vi "ReversedEngineering SortTypeDefsInOrder.vi"(1 "Types":T1(array[cluster])) -> (15 "TypesOut":T1(array[cluster]))   [LabVIEW 2016]
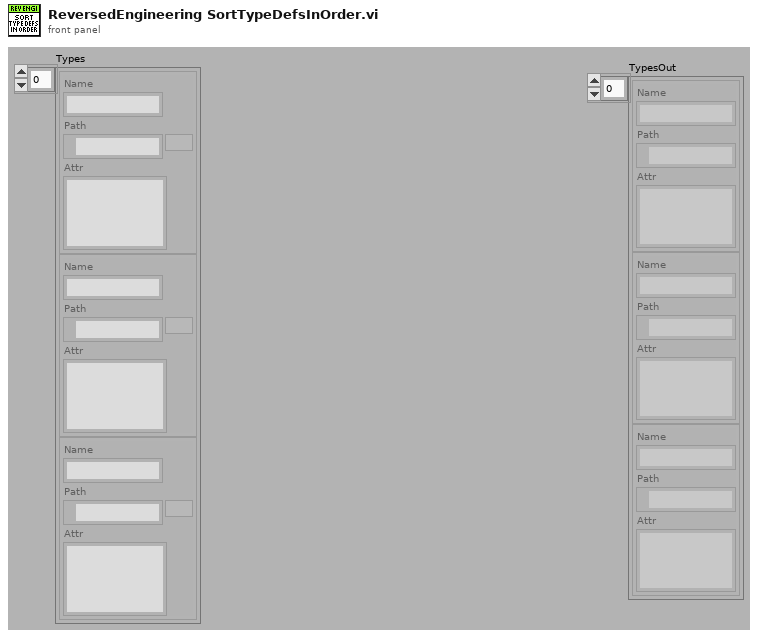
[diagram p1: front panel]
types:
  T1 = cluster{"Name":string, "Path":path, "Attr":string}[]
  T2 = cluster{"Name":string, "Path":path, "Attr":string}
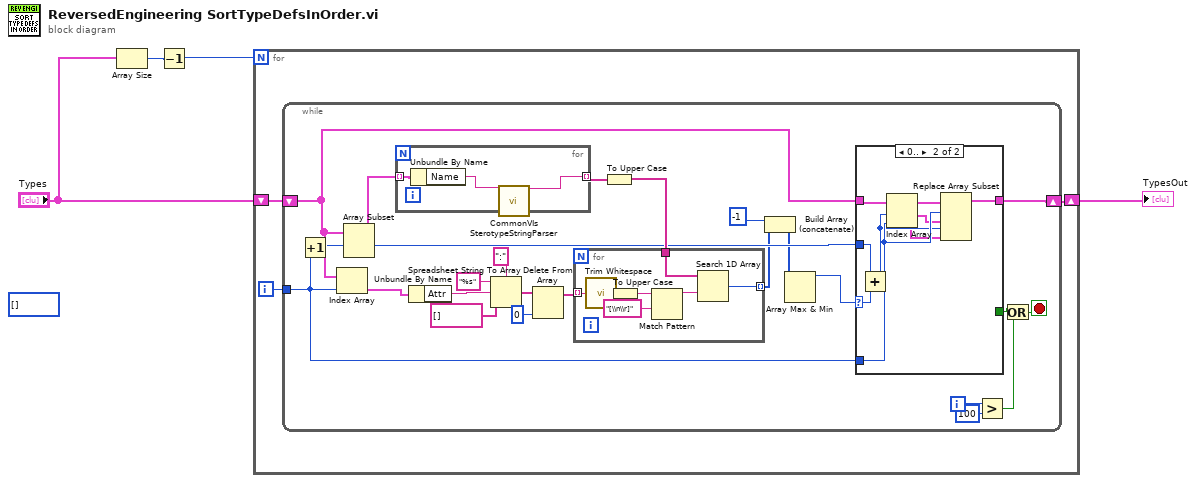
[diagram p0: block diagram]
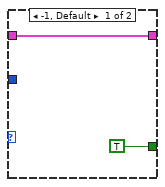
[diagram p2: hidden frame]
diagram:
  (unwired) i32[] []
  n1 = Array Size(array="Types") -> (size(s)=w2:i32)
  n2 = Decrement(x=w2) -> (x-1=w1:i32)
  n3 = for {
    N: w1 -> [_]
    shift-right: [w5] -> w4
    shift-left: "Types" -> [w6]
    i -> [w7]
    n4 = while {
      tunnel: w7 -> [w13]
      shift-right: [w20] -> w5
      shift-left: w6 -> [w19]
      i -> [w17]
      stop <- w15 stop-if-true
      n5 = Increment(x=w13) -> (x+1=w12:i32)
      n6 = Index Array(array=w19, index=w13) -> (element=w21:T2)
      n7 = Array Subset(array=w19, index=w12) -> (w22:T1)  [unwired: 1 in]
      n8 = for {
        tunnel: w22 -> [w44] mode=indexing
        tunnel: [w42] -> w27 mode=indexing
        n9 = Unbundle By Name(w44) -> ("Name"=w43:string)
        n10 = call <resource>:"CommonVIs SterotypeStringParser.vi"("SterotypeStringIn"=w43) -> ("Name"=w42:string)  [unwired: 18 out]
      }
      n11 = Unbundle By Name(w21) -> ("Attr"=w31:string)
      n12 = Spreadsheet String To Array(delimiter (Tab)=":", format string="%s", spreadsheet string=w31, array type (2D Dbl)=string[] []) -> (array=w25:string[])
      n13 = Delete From Array(array=w25, index=0) -> (array with subset deleted=w24:string[])  [unwired: 1 in, 1 out]
      n14 = To Upper Case(1:w27) -> (0:w26:string[])
      n15 = for {
        tunnel: w24 -> [w51] mode=indexing
        tunnel: w26 -> [w47]
        tunnel: [w45] -> w9 mode=indexing
        n16 = call <vilib>:"Trim Whitespace.vi"("string"=w51) -> ("trimmed string"=w46:string)  [unwired: 1 in]
        n17 = To Upper Case(1:w46) -> (0:w50:string)
        n18 = Match Pattern(string=w50, regular expression="[\\n\\r]") -> (before substring=w48:string)  [unwired: 4 out]
        n19 = Search 1D Array(1D array=w47, element=w48) -> (index of element=w45:i32)  [unwired: 1 out]
      }
      n20 = Build Array (concatenate)(-1 ("index"), w9) -> (w10:i32[])
      n21 = Array Max & Min(array=w10) -> (max value=w11:i32)  [unwired: 3 out]
      n22 = case shown="0.." w11 {
        selector: w11 -> [_ w39]
        tunnel: w19 -> [w33 w41]
        tunnel: [w33 w38] -> w20
        tunnel: w13 -> [_ w40]
        tunnel: [TRUE _] -> w18
        tunnel: w12 -> [_ w34]
        frame -1, Default {
        }
        frame 0.. {
          n23 = Add(x=w34, y=w39) -> (x+y=w37:i32)
          n24 = Index Array(array=w41, index #1=w37, index #2=w40) -> (element #1=w36:T2, element #2=w35:T2)
          n25 = Replace Array Subset(array=w41, new element #1=w36, index #1=w40, new element #2=w35, index #2=w37) -> (w38:T1)
        }
      }
      n26 = Greater?(x=w17, y=100) -> (0:w14:bool)
      n27 = Or(x=w18, y=w14) -> (x .or. y?=w15:bool)
    }
  }
  "TypesOut" <- w4
